vi "BufferedAverageFilter_w_StdDev.vi"(7 "Buffer Size":i32, 11 "Signal":dbl) -> (3 "FilteredSignal":dbl, 5 "standard deviation":dbl format="%0.2f")   [LabVIEW 2018]
doc: "Simple Low-Pass filter.\nAverages the last N samples."
uses:
  <vilib>/Analysis/NI_AALBase.lvlib
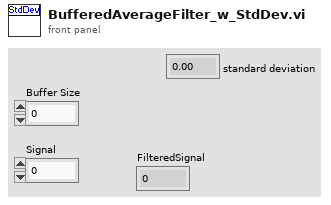
[diagram p1: front panel]
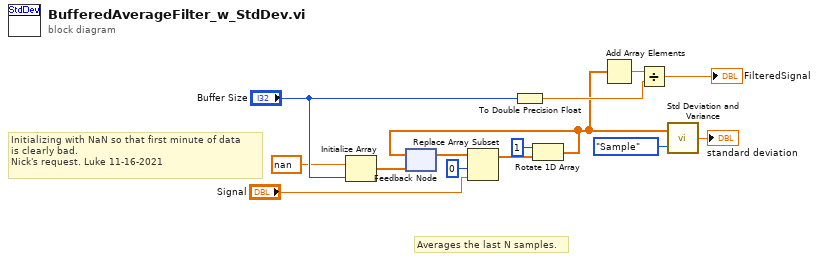
[diagram p0: block diagram]
diagram:
  # "Initializing with NaN so that first minute of data\nis clearly bad. \nNick's request. Luke 11-16-2021"
  # "Averages the last N samples."
  n1 = Initialize Array(nan ("element"), "Buffer Size") -> (w8:dbl[])
  n2 = feedback #1(w8) -> (w10:dbl[])
  n3 = Replace Array Subset(array=w10, new element="Signal", index=0) -> (w11:dbl[])
  n4 = To Double Precision Float(number="Buffer Size") -> (double precision float=w7:dbl)
  n5 = Rotate 1D Array(1:w11, 2:1 ("n")) -> (0:w5:dbl[])
  n6 = feedback-in #1(w5) -> ()
  n7 = Add Array Elements(numeric array=w5) -> (sum=w13:dbl)
  n8 = Divide(x=w13, y=w7) -> (x/y=→"FilteredSignal":dbl)
  n9 = call <vilib>:"Std Deviation and Variance.vi"("X"=w5, "Weighting (Sample)"=enum16{"Sample", "Population"}."Sample") -> ("standard deviation"=→"standard deviation":dbl)  [unwired: 2 out]
